vi "Copy Image To LV.vi"(8 "error in (no error)":errorcluster, 11 "buff":string) -> (0 "error out":errorcluster, 2 "function return":i32, 3 "buff out":string)   [LabVIEW 2017, in "BonTechWrapperLibrary.lvlib"]
doc: "extern \"C\" BONTECHLIBRARY_API int __stdcall CopyImageToLV(char* buff);"
uses:
  BonTechWrapperLibrary.lvlib
  BonTechWrapperLibrary.dll
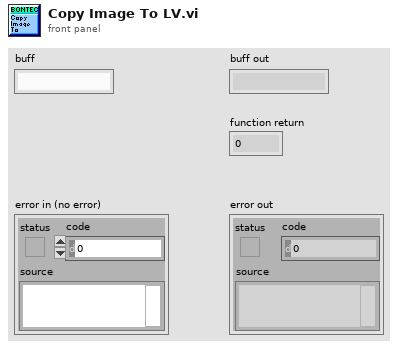
[diagram p1: front panel]
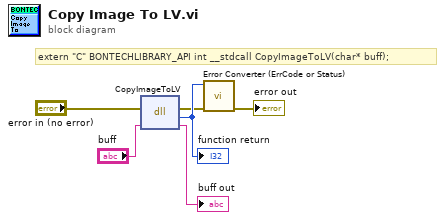
[diagram p0: block diagram]
diagram:
  # "extern \"C\" BONTECHLIBRARY_API int __stdcall CopyImageToLV(char* buff);"
  n1 = dll-call lib="C:/Users/Achuthaperumal/SourceCodes/BonTechWrapperLibrary/BonTechWrapperLibrary/x64/Release/BonTechWrapperLibrary.*" fn="CopyImageToLV"(error in="error in (no error)", "buff"="buff") -> (error out=w2:errorcluster, w6:i32, "buff"=→"buff out":string)  [unwired: 2 in, 1 out]
  "function return" <- w6
  n2 = call "Error Converter (ErrCode or Status).vi"("error in (no error)"=w2, "error code"=w6) -> ("error out"=→"error out":errorcluster)  [unwired: 9 in]
